vi "Setup treatment.vi"(4 "Noise":dbl min=0.0 step=0.5, 5 "End freq":dbl=1.0 min=0.0 step=0.05, 6 "Amplitude":dbl=30.0 min=0.0 step=1.0, 7 "Frequency":dbl=1.0 min=0.0 step=0.05, 8 "Duration unit":enum16{"sec", "cycles"}(ring)=enum."cycles", 9 "Duration":dbl=inf min=0.0 step=1.0, 10 "Treatment type":T1, 11 "Current treatment in":T2) -> (3 "Current treatment out":T2)   [LabVIEW 2012]
uses:
  Treatment.ctl
  Treatment type.ctl
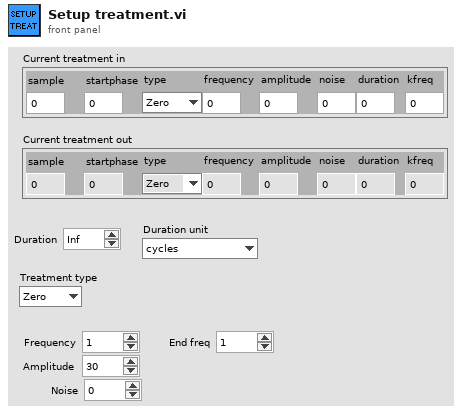
[diagram p1: front panel]
types:
  T1 = typedef "Treatment type.ctl" = enum16{"Zero", "Sine", "Frequency sweep"}
  T2 = typedef "Treatment.ctl" = cluster{"sample":dbl, "startphase":dbl, "type":T1, "frequency":dbl, "amplitude":dbl, "noise":dbl, "duration":dbl, "kfreq":dbl}
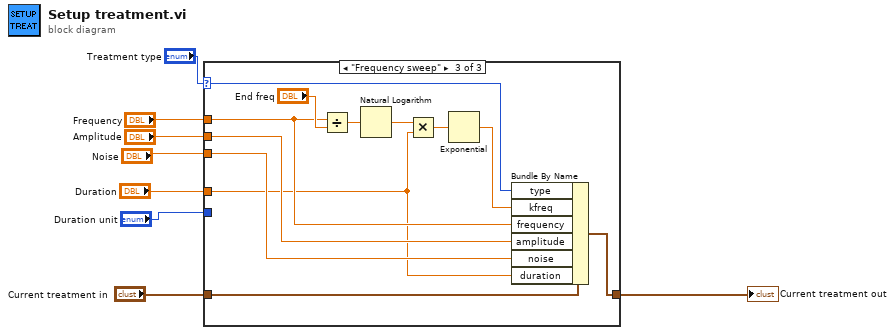
[diagram p0: block diagram]
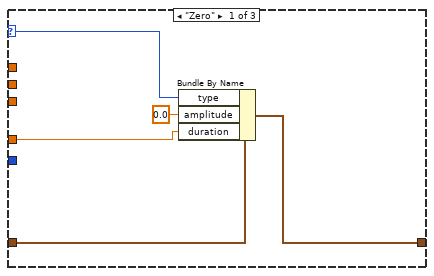
[diagram p2: hidden frame]
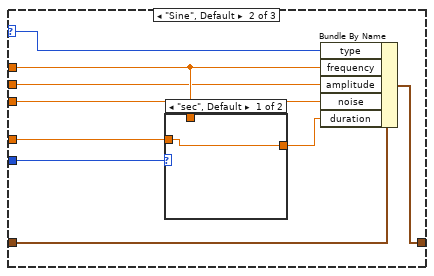
[diagram p3: hidden frame]
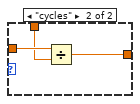
[diagram p4: hidden frame]
diagram:
  n1 = case shown="\"Frequency sweep\"" "Treatment type" {
    selector: "Treatment type" -> [w13 w17 w29]
    tunnel: "Current treatment in" -> [w10 w22 w27]
    tunnel: [w9 w21 w28] -> w8
    tunnel: "Duration unit" -> [_ w20 _]
    tunnel: "Duration" -> [w11 w19 w31]
    tunnel: "Frequency" -> [_ w16 w34]
    tunnel: "Amplitude" -> [_ w15 w33]
    tunnel: "Noise" -> [_ w14 w32]
    frame "Zero" {
      n2 = Bundle By Name(cluster=w10, "type"=w13, "amplitude"=0.0, "duration"=w11) -> (w9:T2)
    }
    frame "Sine", Default {
      n3 = case shown="\"sec\", Default" w20 {
        tunnel: w19 -> [w23 w26]
        tunnel: w16 -> [_ w25]
        tunnel: [w23 w24] -> w18
        frame "sec", Default {
        }
        frame "cycles" {
          n4 = Divide(x=w26, y=w25) -> (x/y=w24:dbl)
        }
      }
      n5 = Bundle By Name(cluster=w22, "type"=w17, "frequency"=w16, "amplitude"=w15, "noise"=w14, "duration"=w18) -> (w21:T2)
    }
    frame "Frequency sweep" {
      n6 = Divide(x=w34, y="End freq") -> (x/y=w37:dbl)
      n7 = Natural Logarithm(1:w37) -> (0:w36:dbl)
      n8 = Multiply(x=w36, y=w31) -> (x*y=w35:dbl)
      n9 = Exponential(1:w35) -> (0:w30:dbl)
      n10 = Bundle By Name(cluster=w27, "type"=w29, "kfreq"=w30, "frequency"=w34, "amplitude"=w33, "noise"=w32, "duration"=w31) -> (w28:T2)
    }
  }
  "Current treatment out" <- w8
